vi "NF LI56xx dvr OPC.vi"(8 "error in":errorcluster caption="error in (no error)" {"code" format="%.0x"}, 9 "Read(F)":bool, 11 "VISA resource name":refnum<visa-resource-name>) -> (0 "error out":errorcluster {"code" format="%.0x"}, 3 "VISA resource name copy":refnum<visa-resource-name>)   [LabVIEW 2019]
doc: "Verifies that execution of all preceding commands has been completed."
panel:
  out "OPC bit":bool
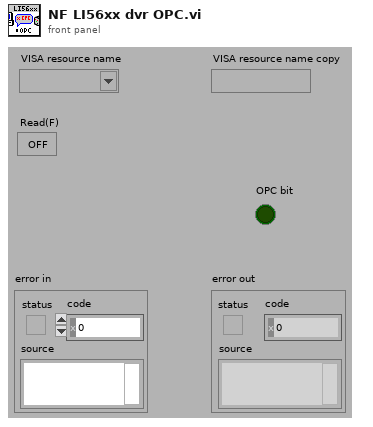
[diagram p1: front panel]
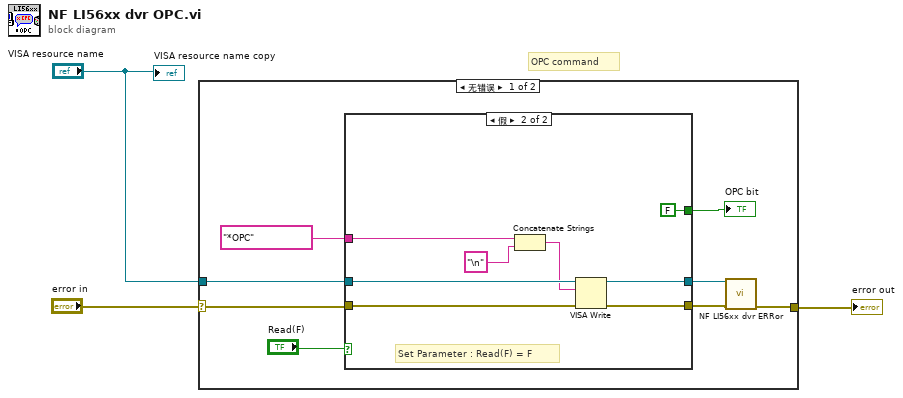
[diagram p0: block diagram]
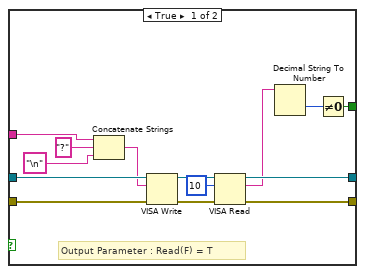
[diagram p2: hidden frame]
diagram:
  # "OPC command"
  n1 = case shown="无错误" "error in" {
    selector: "error in" -> [w10 w34]
    tunnel: [w6 w34] -> w3
    tunnel: "VISA resource name" -> [w9 _]
    frame No Error {
      n2 = case shown="假" "Read(F)" {
        tunnel: w9 -> [w25 w33]
        tunnel: [w22 w30] -> w8
        tunnel: [w21 w31] -> w7
        tunnel: w10 -> [w20 w32]
        tunnel: "*OPC" ("•¶Žš—ñ") -> [w15 w28]
        tunnel: [w12 FALSE] -> w4
        frame True {
          # "Output Parameter : Read(F) = T"
          n3 = Concatenate Strings(w15, "?" ("Œ`Ž®•¶Žš—ñ"), "\n" ("Œ`Ž®•¶Žš—ñ")) -> (w17:string)
          n4 = VISA Write(VISA resource name=w25, write buffer=w17, error in (no error)=w20) -> (VISA resource name out=w23:refnum<visa-resource-name>, error out=w24:errorcluster)  [unwired: 1 out]
          n5 = VISA Read(VISA resource name=w23, byte count=u32 10 ("バイトカウント（0）"), error in (no error)=w24) -> (VISA resource name out=w22:refnum<visa-resource-name>, read buffer=w13:string, error out=w21:errorcluster)  [unwired: 1 out]
          n6 = Decimal String To Number(string=w13) -> (number=w14:i32)  [unwired: 2 in, 1 out]
          n7 = Not Equal To 0?(x=w14) -> (x != 0?=w12:bool)
        }
        frame False {
          # "Set Parameter : Read(F) = F"
          n8 = Concatenate Strings(w28, "\n" ("Œ`Ž®•¶Žš—ñ")) -> (w29:string)
          n9 = VISA Write(VISA resource name=w33, write buffer=w29, error in (no error)=w32) -> (VISA resource name out=w30:refnum<visa-resource-name>, error out=w31:errorcluster)  [unwired: 1 out]
        }
      }
      "OPC bit" <- w4
      n10 = call "NF LI56xx dvr ERRor.vi"("VISA resource name"=w8, "error in (no error)"=w7) -> ("error out"=w6:errorcluster)  [unwired: 10 in, 3 out]
    }
    frame Error {
    }
  }
  "error out" <- w3
  "VISA resource name copy" <- "VISA resource name"
